vi "gyro -- launch async vi -- V1.vi"(6 "VI Refnum":refnum<vi>, 11 "pll event pair IN":T1) -> (2 "reference out":refnum<vi>, 3 "pll event pair OUT":T1)   [LabVIEW 2021]
uses:
  server talk-to-back pair.ctl
  server talkback message type.ctl
  server talkto message type.ctl
panel:
  in  "set step !":dbl(slide)=7372.340425531916 min=0.0 max=16000.0 scale=0.0..16500.0 scale format="%^#6_6g"
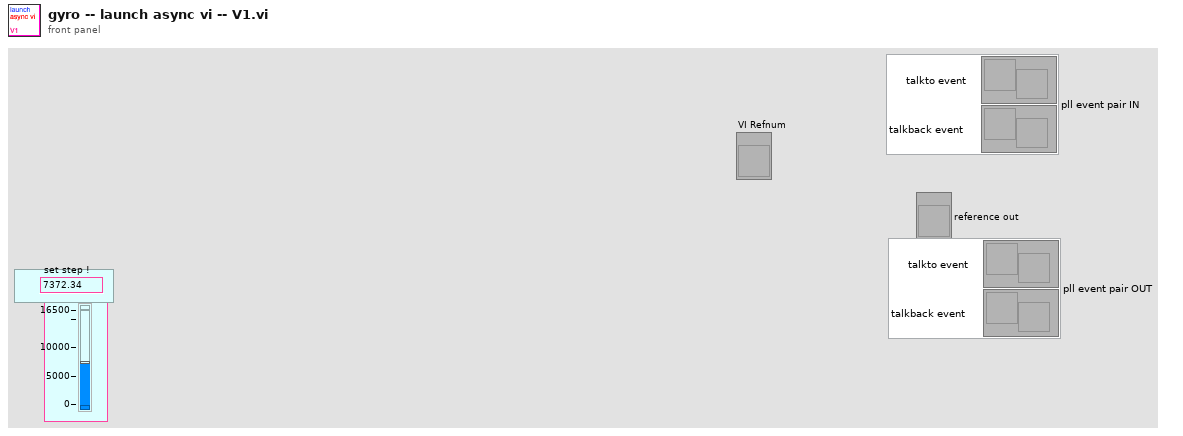
[diagram p1: front panel]
types:
  T1 = typedef "server talk-to-back pair.ctl" = cluster{"talkback event":refnum<user-event>, "talkto event":refnum<user-event>}
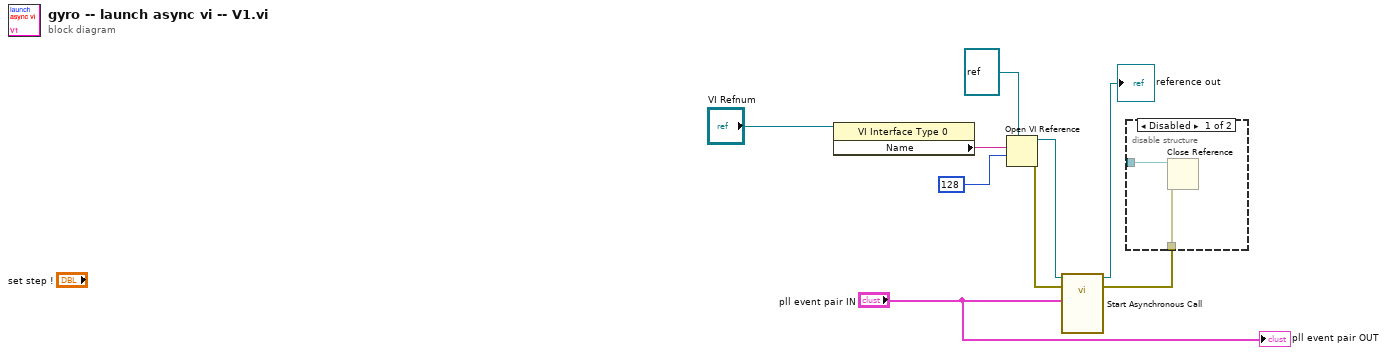
[diagram p0: block diagram]
diagram:
  n1 = property class="VI Interface Type 0"(reference="VI Refnum") -> ("Name"=w8:string)  [unwired: 1 in, 2 out]
  n2 = Open VI Reference(type specifier VI Refnum (for type only)=refnum<vi> refnum, vi path=w8, options=128) -> (vi reference=w4:refnum<vi>, error out=w3:errorcluster)  [unwired: 3 in]
  n3 = call-by-ref "Start Asynchronous Call"(reference=w4, error in=w3, "pll event pair"="pll event pair IN") -> (reference out=→"reference out":refnum<vi>, error out=w6:errorcluster)  [unwired: 11 in]
  n4 = disable-structure shown="Disabled" {
    disable-tunnel: w6 -> [w11 _]
    disable-tunnel: _ -> [w10 _]
    frame Disabled {
      n5 = Close Reference(reference=w10, error in (no error)=w11) -> ()  [unwired: 1 out]
    }
    frame Enabled {
    }
  }
  "pll event pair OUT" <- "pll event pair IN"
